vi "Get Num of Sheets.vi"(8 "error in (no error)":errorcluster, 11 "List_UI in":refnum<class "List_UI.lvclass">) -> (0 "error out":errorcluster, 2 "NumOfSheets":i32, 3 "List_UI out":refnum<class "List_UI.lvclass">)   [LabVIEW 2015, in "List_UI.lvclass"]
uses:
  List_UI.lvclass
  List_UI.lvclass/List_UI.ctl
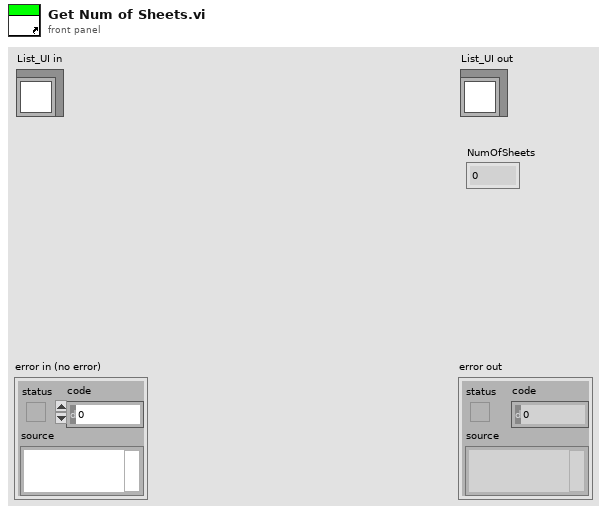
[diagram p1: front panel]
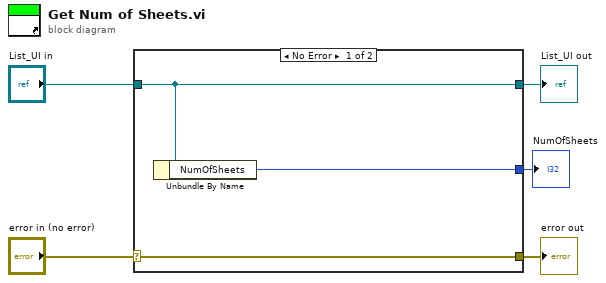
[diagram p0: block diagram]
diagram:
  n1 = case shown="No Error" "error in (no error)" {
    selector: "error in (no error)" -> [w8 w9]
    tunnel: [w8 w9] -> w4
    tunnel: [w7 w10] -> w2
    tunnel: "List_UI in" -> [w7 w10]
    tunnel: [w6 _] -> w1
    frame No Error {
      n2 = Unbundle By Name(w7) -> ("NumOfSheets"=w6:i32)
    }
    frame Error {
    }
  }
  "error out" <- w4
  "List_UI out" <- w2
  "NumOfSheets" <- w1
